vi "Set Default.vi"(8 "error in (no error)":errorcluster, 11 "DMM Config RTD Type Msg in":refnum<class "DMM Config RTD Type Msg.lvclass">) -> (0 "error out":errorcluster, 3 "DMM Config RTD Type Msg out":refnum<class "DMM Config RTD Type Msg.lvclass">)   [LabVIEW 2020, in "DMM Msg.lvlib" / "DMM Config RTD Type Msg.lvclass"]
doc: "Restore private data to a defined default state.\n\nThis implementation sets:\nPt3851 with 100 Ohms at 0°C.\nAwait reply, -1ms timeout at normal priority without publish."
uses:
  DMM Config RTD Type Msg.lvclass
  PPL/HDH.Actor Framework.Core.Actor.lvlibp/1abvi3w/vi.lib/ActorFramework/Message Enqueuer/Message Priority.ctl
  PPL/HDH.Actor Framework.Core.Publisher.lvlibp/Messages/Response Msg/Response Core/Controls/Ctl_SendFunction.ctl
  PPL/HDH.Driver.DMM.lvlibp/Controls/Ctl_RTDType.ctl
  DMM Config RTD Type Msg.lvclass/DMM Config RTD Type Msg.ctl
  DMM Msg/DMM Msg.lvclass
  PPL/HDH.Driver.DMM.lvlibp
  PPL/HDH.Actor Framework.Core.Instrument Handler.lvlibp/Messages/Instrument Msg/Instrument Msg.lvclass
  PPL/HDH.Actor Framework.Core.Publisher.lvlibp
  PPL/HDH.Actor Framework.Core.Actor.lvlibp/1abvi3w/vi.lib/ActorFramework/Message Enqueuer/Message Enqueuer.lvclass
  C:/Current projects/WS/PPL/HDH.Actor Framework.Core.Instrument Handler.lvlibp/Messages/Instrument Msg/Instrument Msg.lvclass
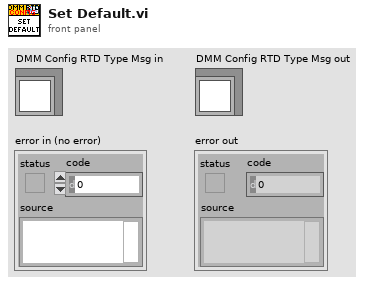
[diagram p1: front panel]
types:
  T1 = typedef "HDH.Driver.DMM.lvlibp/Ctl_RTDType.ctl" = enum16{"Custom", "Pt3750", "Pt3851", "Pt3911", "Pt3916", "Pt3920", "Pt3928"}
  T2 = typedef "HDH.Actor Framework.Core.Publisher.lvlibp/Ctl_SendFunction.ctl" = enum16{"Send and Forget", "Request Reply", "Await Reply"}
  T3 = typedef "HDH.Actor Framework.Core.Actor.lvlibp/Message Enqueuer.lvclass/Message Priority.ctl" = enum16{"Low", "Normal", "High"}
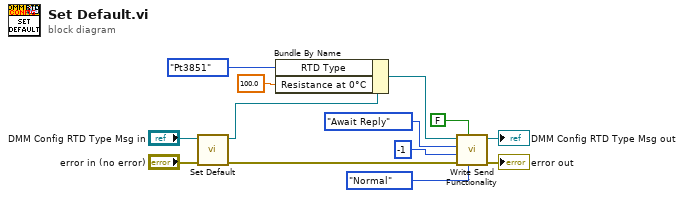
[diagram p0: block diagram]
diagram:
  n1 = call-parent "Set Default.vi"("error in (no error)"="error in (no error)", "Flex Msg in"="DMM Config RTD Type Msg in") -> ("error out"=w7:errorcluster, "Flex Msg out"=w13:refnum<class "DMM Config RTD Type Msg.lvclass">)  [unwired: 8 in]
  n2 = Bundle By Name(cluster=w13, "RTD Type"=Ctl_RTDType."Pt3851", "Resistance at 0°C"=100.0) -> (w10:refnum<class "DMM Config RTD Type Msg.lvclass">)
  n3 = call "Write Send Functionality.vi"("Message Priority(Normal)"=Message_Priority."Normal", "Publish Data?(T)"=FALSE, "error in (no error)"=w7, "Timeout if Waiting(-1ms)"=-1, "Send Function(Await Reply)"=Ctl_SendFunction."Await Reply", "Instrument Msg in"=w10) -> ("error out"=→"error out":errorcluster, "Instrument Msg out"=→"DMM Config RTD Type Msg out":refnum<class "DMM Config RTD Type Msg.lvclass">)  [unwired: 4 in]
